vi "ROS_Master_removeService.vi"(2 "Service":T5, 3 "ROS_Master in":T1) -> (0 "error out":errorcluster, 1 "ROS_Master out":T1)   [LabVIEW 2015]
doc: "Unregisters a service with the master and updates list of services registered to reflect change"
uses:
  ROS_Master.ctl
  ROS_Topic.ctl
  ROS_Node.ctl
  ROS_Service.ctl
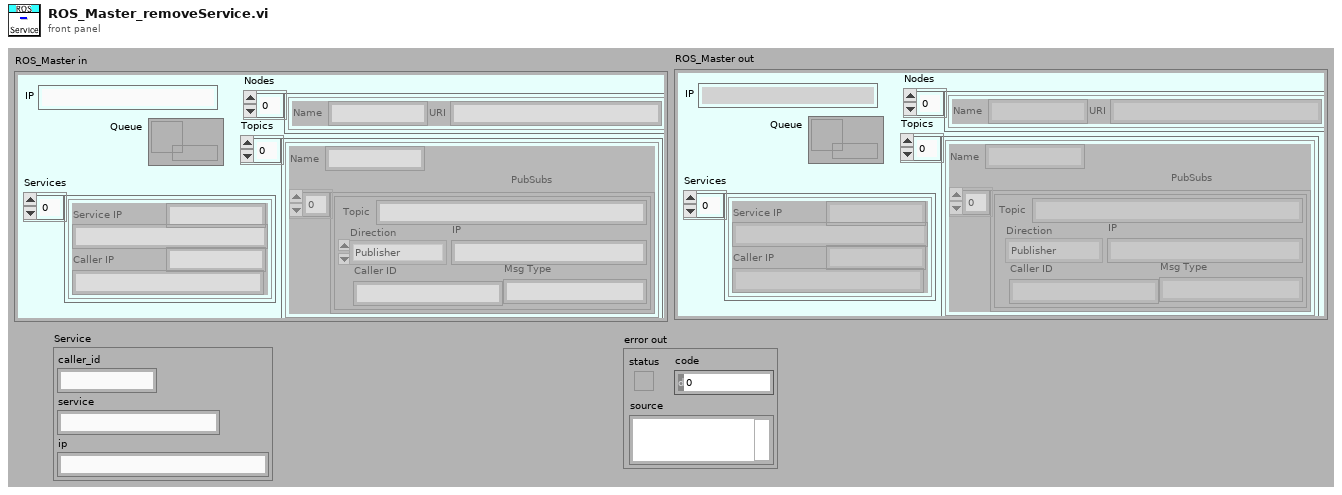
[diagram p1: front panel]
types:
  T1 = typedef "ROS_Master.ctl" = cluster{"IP":string, "Topics":cluster{"Name":string, "PubSubs":T2[]}[], "Nodes":T3[], "Services":T4[], "Queue":refnum<queue>}
  T2 = typedef "ROS_Topic.ctl" = cluster{"Caller ID":string, "IP":string, "Msg Type":string, "Direction":enum16{"Publisher", "Subscriber"}, "Topic":string}
  T3 = typedef "ROS_Node.ctl" = cluster{"Name":string, "URI":string}
  T4 = typedef "ROS_Service.ctl" = cluster{"Service":string, "Service IP":string, "Caller IP":string, "Caller ID":string}
  T5 = cluster{"caller_id":string, "service":string, "ip":string}
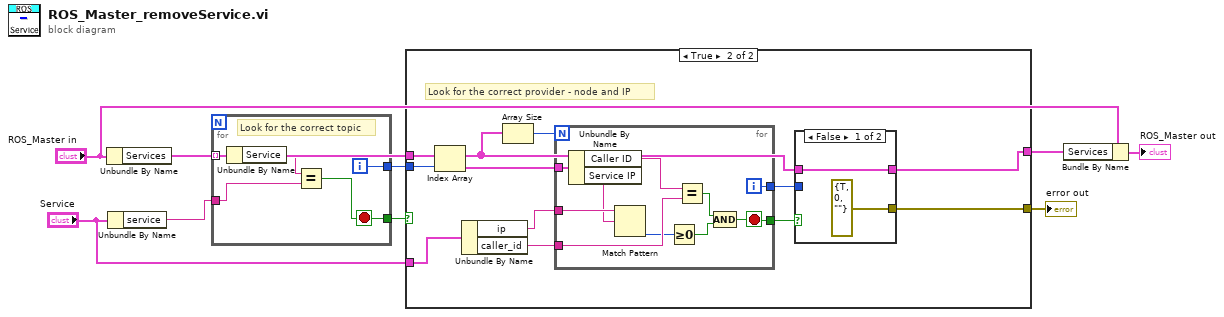
[diagram p0: block diagram]
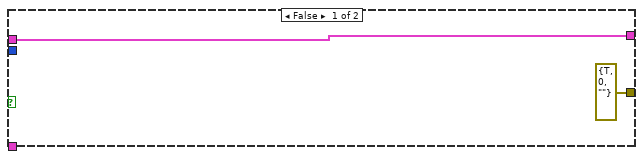
[diagram p2: hidden frame]
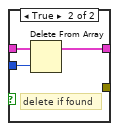
[diagram p3: hidden frame]
diagram:
  n1 = Unbundle By Name("ROS_Master in") -> ("Services"=w8:T4[])
  n2 = Unbundle By Name("Service") -> ("service"=w9:string)
  n3 = for {
    tunnel: w8 -> [w14] mode=indexing
    tunnel: w9 -> [w12]
    tunnel: [w11] -> w7
    tunnel: [w10] -> w6
    i -> [w11]
    stop <- w10 stop-if-true
    # "Look for the correct topic"
    n4 = Unbundle By Name(w14) -> ("Service"=w13:string)
    n5 = Equal?(x=w13, y=w12) -> (x = y?=w10:bool)
  }
  n6 = case shown="True" w6 {
    tunnel: w8 -> [w16 w18]
    tunnel: w7 -> [_ w22]
    tunnel: "Service" -> [_ w27]
    tunnel: [w16 w19] -> w5
    tunnel: [errorcluster {"status"=TRUE, "code"=0, "source"=""} ("error constant") w21] -> w3
    frame False {
    }
    frame True {
      # "Look for the correct provider - node and IP"
      n7 = Index Array(array=w18, index=w22) -> (element=w20:T4)
      n8 = Unbundle By Name(w27) -> ("ip"=w25:string, "caller_id"=w26:string)
      n9 = Array Size(array=w18) -> (size(s)=w17:i32)
      n10 = for {
        N: w17 -> [_]
        tunnel: w20 -> [w42]
        tunnel: w26 -> [w40]
        tunnel: w25 -> [w39]
        tunnel: [w33] -> w24
        tunnel: [w36] -> w23
        i -> [w36]
        stop <- w33 stop-if-true
        n11 = Unbundle By Name(w42) -> ("Caller ID"=w41:string, "Service IP"=w38:string)
        n12 = Match Pattern(string=w39, regular expression=w38) -> (offset past match=w37:i32)  [unwired: 1 in, 3 out]
        n13 = Greater Or Equal To 0?(x=w37) -> (x >= 0?=w35:bool)
        n14 = Equal?(x=w41, y=w40) -> (x = y?=w34:bool)
        n15 = Compound Arithmetic op=AND(w34, w35) -> (w33:bool)
      }
      n16 = case shown="False" w24 {
        tunnel: w18 -> [w29 w32]
        tunnel: w23 -> [_ w31]
        tunnel: [w29 w30] -> w19
        tunnel: [errorcluster {"status"=TRUE, "code"=0, "source"=""} ("error constant") _] -> w21
        frame False {
        }
        frame True {
          # "delete if found"
          n17 = Delete From Array(array=w32, index=w31) -> (array with subset deleted=w30:T4[])  [unwired: 1 in, 1 out]
        }
      }
    }
  }
  "error out" <- w3
  n18 = Bundle By Name(cluster="ROS_Master in", "Services"=w5) -> (→"ROS_Master out":T1)
